vi "DisableEnable.vi"(8 "error in (no error)":errorcluster, 10 "Action":T1(ring)=enum."Disabled and Grayed Out", 11 "Array of Control References":refnum<vi>[](array[refnum])) -> (0 "error out":errorcluster)   [LabVIEW 2024]
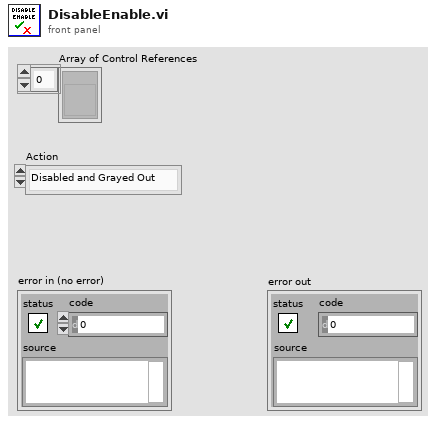
[diagram p1: front panel]
types:
  T1 = enum8{"Enabled", "Disabled", "Disabled and Grayed Out"}
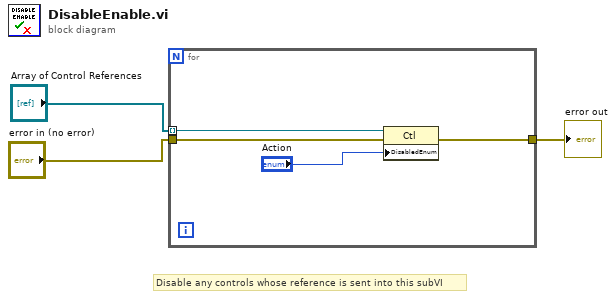
[diagram p0: block diagram]
diagram:
  # "Disable any controls whose reference is sent into this subVI"
  n1 = for {
    tunnel: "Array of Control References" -> [w7] mode=indexing
    tunnel: [w5] -> w3
    tunnel: "error in (no error)" -> [w4]
    n2 = property class="Ctl"(reference=w7, error in=w4, "DisabledEnum"="Action") -> (error out=w5:errorcluster)  [unwired: 1 out]
  }
  "error out" <- w3
